vi "HarvestPips.vi"(6 "Stop on 1st fail":bool, 7 "Banana":refnum<class "Banana.lvclass">, 8 "error in (no error)":errorcluster, 11 "Pips":refnum<class "Pips.lvclass">) -> (0 "error out":errorcluster, 3 "Pips":refnum<class "Pips.lvclass">)   [LabVIEW 2021, in "Bananas.lvlib" / "Platano.lvclass"]
uses:
  Platano.lvclass
  Banana/Banana.lvclass
  BananaPeel/BananaPeel.lvclass
  Pips/Pips.lvclass
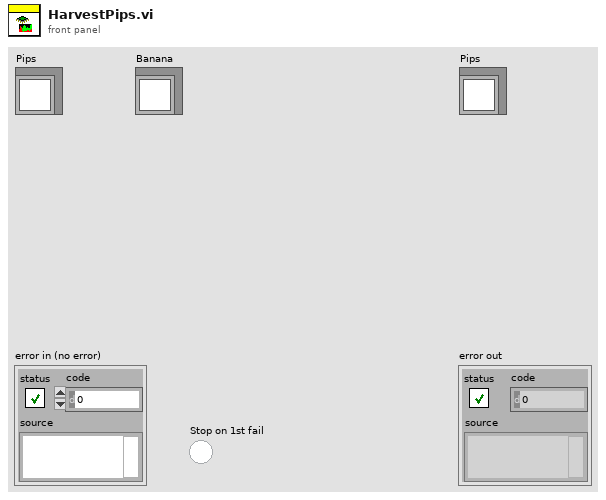
[diagram p1: front panel]
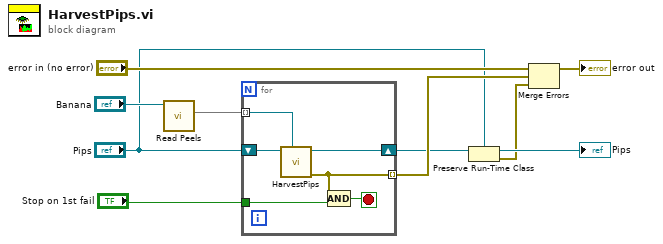
[diagram p0: block diagram]
diagram:
  n1 = call "Read Peels.vi"("Banana in"="Banana") -> ("Peels"=w5:set{refnum<class "BananaPeel.lvclass">})  [unwired: 8 in, 2 out]
  n2 = for {
    tunnel: [w11] -> w10 mode=indexing
    shift-right: [w12] -> w4
    shift-left: "Pips" -> [w13]
    tunnel: w5 -> [w14] mode=indexing
    tunnel: "Stop on 1st fail" -> [w16]
    stop <- w15 stop-if-true
    n3 = call "HarvestPips.vi"("BananaPeel in"=w14, "Pips"=w13) -> ("error out"=w11:errorcluster, "Pips"=w12:refnum<class "Pips.lvclass">)  [unwired: 8 in]
    n4 = Compound Arithmetic op=AND(w11, w16) -> (w15:bool)
  }
  n5 = Preserve Run-Time Class(object in=w4, 2:"Pips") -> (object out=→"Pips":refnum<class "Pips.lvclass">, error out=w1:errorcluster)  [unwired: 1 in]
  n6 = Merge Errors("error in (no error)", w10, w1) -> (→"error out":errorcluster)
